vi "RuO2 2k.vi"(1 "temperature \n(OR resistance)":dbl) -> (0 "resistance \n(OR temperature)":dbl)   [LabVIEW 2013]
panel:
  # "This tool convert data for a 2K thermometer (RuO2). Edit \nconstants in the block diagram to modify calibration."
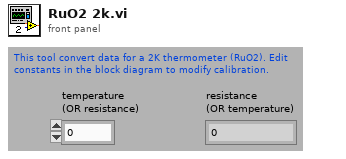
[diagram p1: front panel]
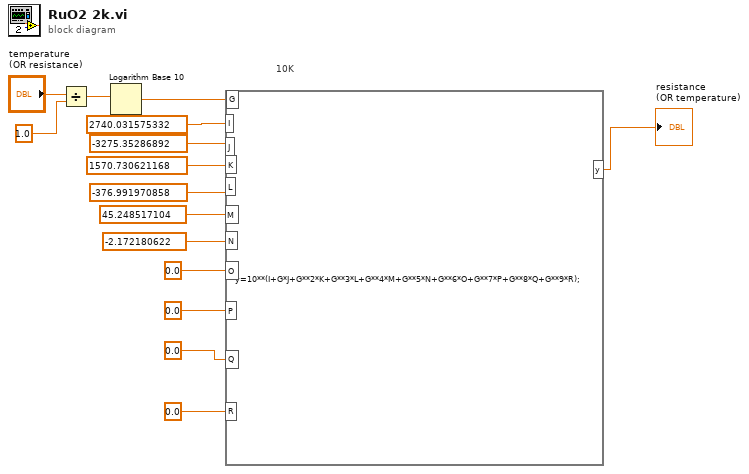
[diagram p0: block diagram]
diagram:
  # "10K"
  n1 = Divide(x="temperature \n(OR resistance)", y=1.0) -> (x/y=w2:dbl)
  n2 = Logarithm Base 10(1:w2) -> (0:w15:dbl)
  n3 = formula code="y=10**(I+G*J+G**2*K+G**3*L+G**4*M+G**5*N+G**6*O+G**7*P+G**8*Q+G**9*R);"("G"=w15, "I"=2740.031575332 ("input variable"), "L"=-376.991970858 ("input variable"), "M"=45.248517104 ("input variable"), "O"=0.0 ("input variable"), "Q"=0.0 ("input variable"), "R"=0.0 ("input variable"), "P"=0.0 ("input variable"), "N"=-2.172180622 ("input variable"), "J"=-3275.35286892 ("input variable"), "K"=1570.730621168 ("input variable")) -> ("y"=→"resistance \n(OR temperature)":dbl)
